vi "SetRamp.vi"(8 "error in (no error)":errorcluster, 11 "VISA Refnum in":refnum<visa-resource-name>) -> (0 "error in (no error) 2":errorcluster, 3 "VISA Refnum Out":refnum<visa-resource-name>)   [LabVIEW 2023]
panel:
  in  "Cooling Ramp °C/s":dbl=0.167 min=0.0 max=1.0
  in  "Heating Ramp °C/s":dbl=0.167 min=0.0 max=1.0
  in  "Time Base (s)":enum16{"Minutes (60)", "Seconds (1)"}(ring)
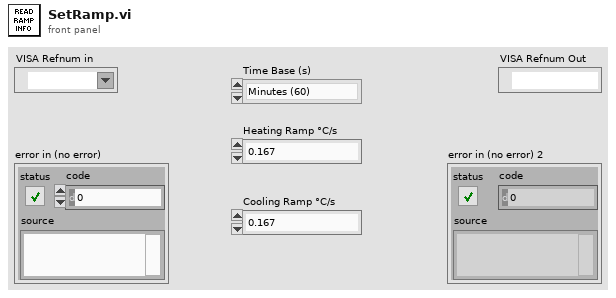
[diagram p1: front panel]
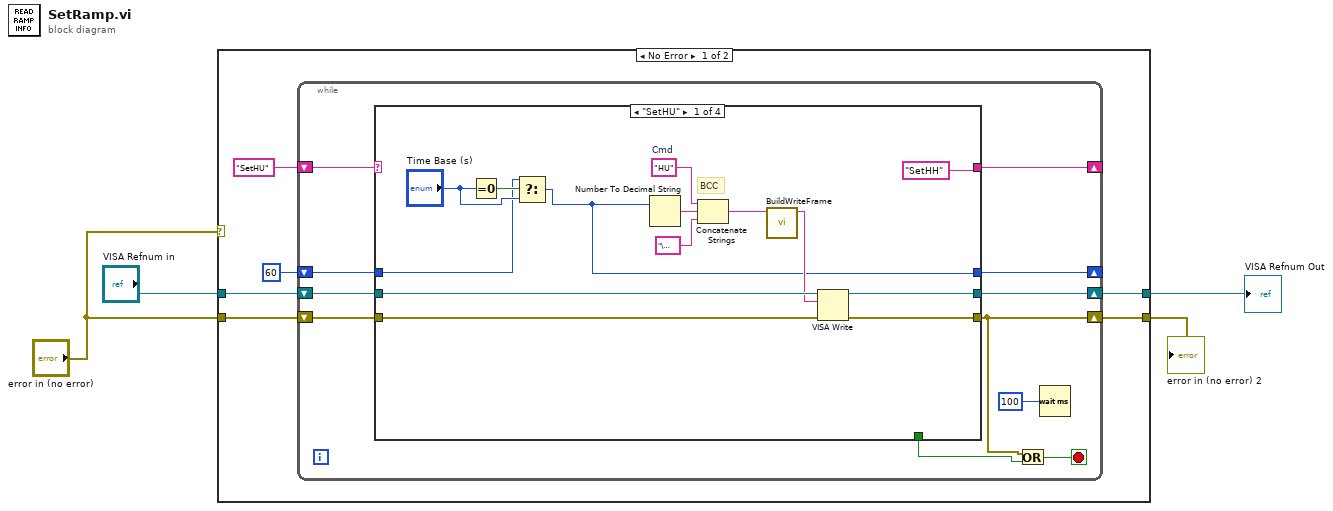
[diagram p0: block diagram]
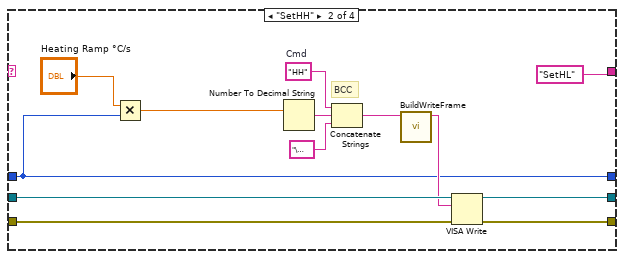
[diagram p2: hidden frame]
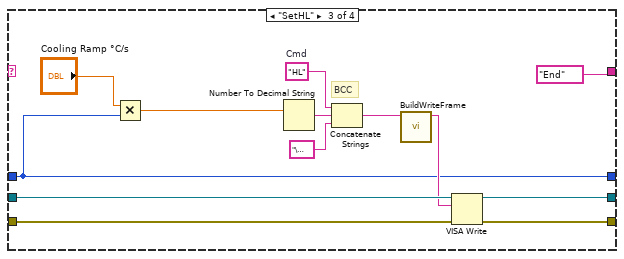
[diagram p3: hidden frame]
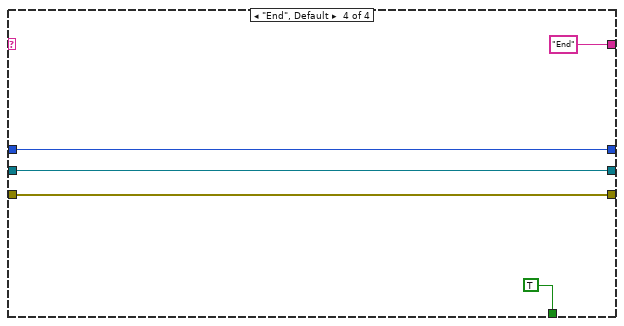
[diagram p4: hidden frame]
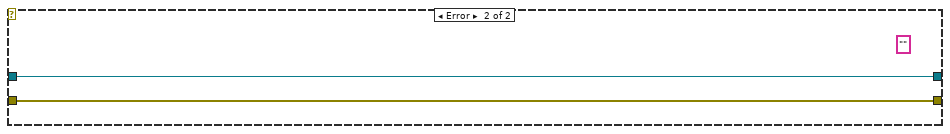
[diagram p5: hidden frame]
diagram:
  n1 = case shown="No Error" "error in (no error)" {
    tunnel: "VISA Refnum in" -> [w10 w68]
    tunnel: "error in (no error)" -> [w9 w67]
    tunnel: [w7 w68] -> w1
    tunnel: [w6 w67] -> w2
    frame No Error {
      n2 = while {
        shift-right: [w18] -> _
        shift-left: "SetHU" -> [w19]
        shift-right: [w13] -> w7
        shift-left: w10 -> [w21]
        shift-right: [w14] -> w6
        shift-left: w9 -> [w20]
        shift-right: [w12] -> _
        shift-left: 60 ("Time Base (s)") -> [w11]
        stop <- w16 stop-if-true
        n3 = case shown="\"SetHU\"" w19 {
          tunnel: w21 -> [w35 w48 w61 w64]
          tunnel: w20 -> [w34 w47 w60 w65]
          tunnel: ["SetHH" "SetHL" "End" "End"] -> w18
          tunnel: [_ _ _ TRUE] -> w15
          tunnel: [w32 w45 w58 w65] -> w14
          tunnel: [w31 w44 w57 w64] -> w13
          tunnel: [w23 w36 w50 w62] -> w12
          tunnel: w11 -> [w22 w36 w50 w62]
          frame "SetHU" {
            w30 = "HU"  # Cmd
            # "BCC"
            n4 = Equal To 0?(x="Time Base (s)") -> (x = 0?=w29:bool)
            n5 = Select(t=w22, s=w29, f="Time Base (s)") -> (s? t:f=w23:i32)
            n6 = Number To Decimal String(number=w23) -> (decimal integer string=w27:string)  [unwired: 1 in]
            n7 = Concatenate Strings(w30, w27, "\u0003" ("string")) -> (w25:string)
            n8 = call "BuildWriteFrame.vi"("String in"=w25) -> ("String out"=w24:string)  [unwired: 10 in]
            n9 = VISA Write(VISA resource name=w35, write buffer=w24, error in (no error)=w34) -> (VISA resource name out=w31:refnum<visa-resource-name>, error out=w32:errorcluster)  [unwired: 1 out]
          }
          frame "SetHH" {
            w43 = "HH"  # Cmd
            # "BCC"
            n10 = Multiply(x="Heating Ramp °C/s", y=w36) -> (x*y=w37:dbl)
            n11 = Number To Decimal String(number=w37) -> (decimal integer string=w42:string)  [unwired: 1 in]
            n12 = Concatenate Strings(w43, w42, "\u0003" ("string")) -> (w40:string)
            n13 = call "BuildWriteFrame.vi"("String in"=w40) -> ("String out"=w39:string)  [unwired: 10 in]
            n14 = VISA Write(VISA resource name=w48, write buffer=w39, error in (no error)=w47) -> (VISA resource name out=w44:refnum<visa-resource-name>, error out=w45:errorcluster)  [unwired: 1 out]
          }
          frame "SetHL" {
            w56 = "HL"  # Cmd
            # "BCC"
            n15 = Multiply(x="Cooling Ramp °C/s", y=w50) -> (x*y=w51:dbl)
            n16 = Number To Decimal String(number=w51) -> (decimal integer string=w55:string)  [unwired: 1 in]
            n17 = Concatenate Strings(w56, w55, "\u0003" ("string")) -> (w53:string)
            n18 = call "BuildWriteFrame.vi"("String in"=w53) -> ("String out"=w52:string)  [unwired: 10 in]
            n19 = VISA Write(VISA resource name=w61, write buffer=w52, error in (no error)=w60) -> (VISA resource name out=w57:refnum<visa-resource-name>, error out=w58:errorcluster)  [unwired: 1 out]
          }
          frame "End", Default {
          }
        }
        n20 = Or(x=w14, y=w15) -> (x .or. y?=w16:bool)
        n21 = Wait (ms)(milliseconds to wait=u32 100) -> ()  [unwired: 1 out]
      }
    }
    frame Error {
      (unwired) "" ("read buffer")
    }
  }
  "VISA Refnum Out" <- w1
  "error in (no error) 2" <- w2
